vi "GOOP_ToolVersion.vi"() -> ()   [LabVIEW 2020]
panel:
  in  "Build":string="29"
  in  "Branch":string="Master"
  in  "Version":string="2.5.2"
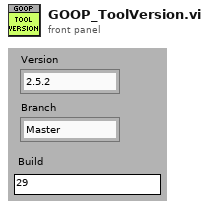
[diagram p1: front panel]
diagram:
